vi "Update.vi"(8 "error in (no error)":errorcluster, 9 "Value":variant, 10 "Key":variant, 11 "Store in":refnum<class "Store.lvclass">) -> (0 "error out":errorcluster, 1 "Success?":bool, 3 "Store out":refnum<class "Store.lvclass">)   [LabVIEW 2018, in "Application.lvlib" / "Store.lvclass"]
uses:
  Store.lvclass
  Store.lvclass/Store.ctl
  Dictionary Class/Dictionary.lvclass/Dictionary.ctl
  4e27f25c-ebf7-46df-ab82-df9d0c9e0099.vi
  Variant to Packed String.vi
  Dictionary Class/VIs/Get Data DVR.vi
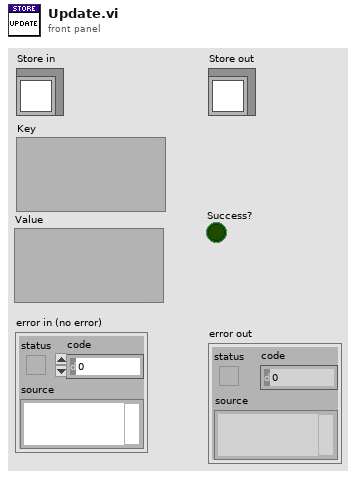
[diagram p1: front panel]
types:
  T1 = typedef "Application.lvlib/Store.lvclass/Packet.ctl" = cluster{"Type Descriptor":i16[], "Value":variant}
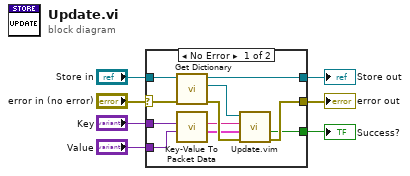
[diagram p0: block diagram]
diagram:
  n1 = case shown="No Error" "error in (no error)" {
    selector: "error in (no error)" -> [w14 w20]
    tunnel: [w12 w20] -> w6
    tunnel: [w15 w19] -> w4
    tunnel: "Store in" -> [w18 w19]
    tunnel: "Key" -> [w17 _]
    tunnel: "Value" -> [w16 _]
    tunnel: [w11 _] -> w1
    frame No Error {
      n2 = call "Get Dictionary.vi"("error in (no error)"=w14, "Store in"=w18) -> ("error out"=w13:errorcluster, "Dictionary.lvclass"=w10:refnum<class "Dictionary.lvclass">, "Store out"=w15:refnum<class "Store.lvclass">)  [unwired: 7 in]
      n3 = call "Key-Value To Packet Data.vi"("Value"=w16, "Key"=w17) -> ("Packet"=w8:T1, "Packed String"=w9:string)  [unwired: 8 in]
      n4 = call "Update.vim"("error in (no error)"=w13, "Value"=w8, "Key"=w9, "Dictionary in"=w10) -> ("error out"=w12:errorcluster, "Success?"=w11:bool)  [unwired: 5 in, 1 out]
    }
    frame Error {
    }
  }
  "error out" <- w6
  "Store out" <- w4
  "Success?" <- w1
